vi "Dequeue Cmds From Nodes.vi"(6 "Ready For Output?":bool, 7 "NumNodes":u8=1, 8 "error in":errorcluster, 11 "Communication FIFOs":T2) -> (0 "error out":errorcluster, 1 "Cmd Received Valid":bool, 2 "Cmd Received":T1, 5 "Current Node":u8)   [LabVIEW 2014, in "IO Node Logic Template.lvlib"]
uses:
  IO Node Logic Template.lvlib
  Controls/All Nodes Resources.ctl
  Node/Controls/NodeResources FIFOs.ctl
  Node/Controls/Node_Command_Sent.ctl
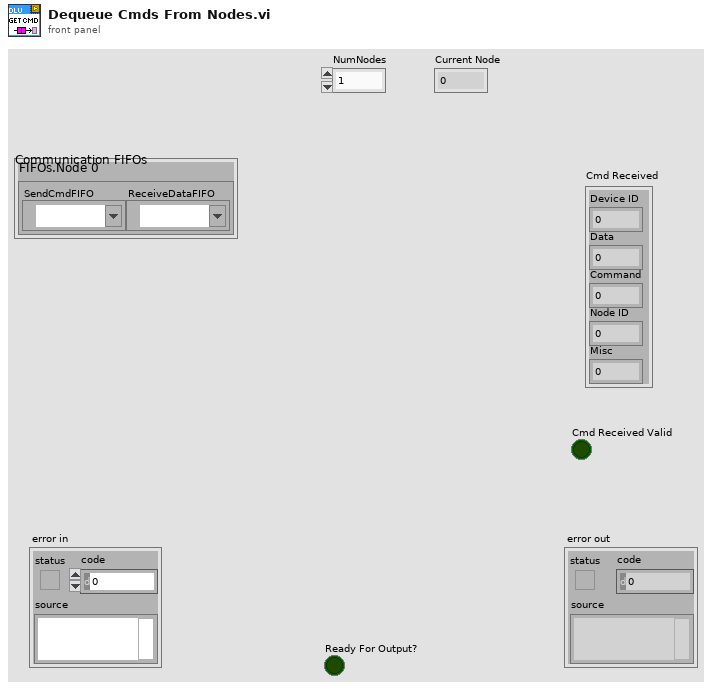
[diagram p1: front panel]
types:
  T1 = typedef "Node_Command_Sent.ctl" = cluster{"Device ID":u8, "Data":u64, "Command":u8, "Node ID":u8, "Misc":u8}
  T2 = typedef "IO Node Logic Template.lvlib/All Nodes Resources.ctl" = cluster{"FIFOs.Node 0":T3}
  T3 = typedef "IO Node Logic Template.lvlib/NodeResources FIFOs.ctl" = cluster{"SendCmdFIFO":refnum<k21>, "ReceiveDataFIFO":refnum<k21>}
  T4 = cluster{"Channel ID":u8, "Data":u64, "Command":u8, "Sender Address":u8, "Misc":u8}
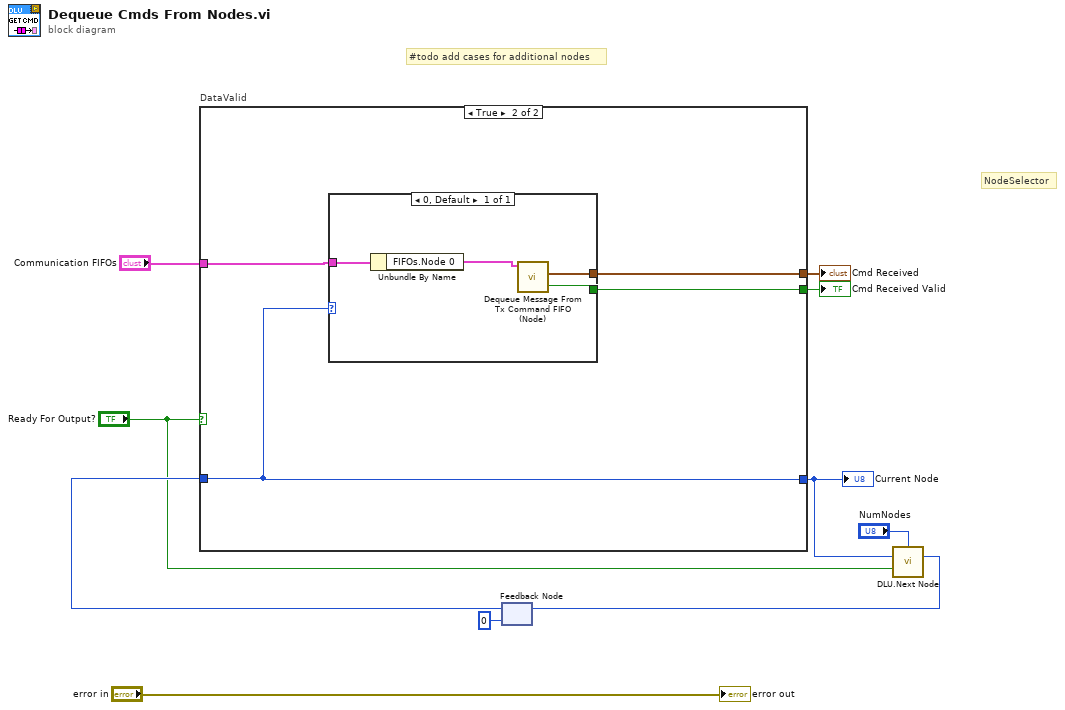
[diagram p0: block diagram]
diagram:
  # "#todo add cases for additional nodes"
  # "NodeSelector"
  n1 = feedback #1(u8 0 ("Next Node")) -> (w7:u8)
  n2 = case "DataValid" shown="True" "Ready For Output?" {
    tunnel: w7 -> [w11 w12]
    tunnel: "Communication FIFOs" -> [_ w15]
    tunnel: [_ w14] -> w3
    tunnel: [_ w13] -> w2
    tunnel: [w11 w12] -> w6
    frame False {
    }
    frame True {
      n3 = case shown="0, Default" w12 {
        tunnel: w15 -> [w19]
        tunnel: [w18] -> w14
        tunnel: [w17] -> w13
        frame 0, Default {
          n4 = Unbundle By Name(w19) -> ("FIFOs.Node 0"=w16:T3)
          n5 = call "Dequeue Message From Tx Command FIFO (Node).vi"("FIFOs: I/O Node"=w16) -> ("Cmd Received Valid"=w17:bool, "Cmd Received"=w18:T4)  [unwired: 7 in, 2 out]
        }
      }
    }
  }
  "Cmd Received" <- w3
  "Cmd Received Valid" <- w2
  "Current Node" <- w6
  n6 = call "DLU.Next Node.vi"("NumNodes"="NumNodes", "Current Node"=w6, "Move to Next Node"="Ready For Output?") -> ("Next Node"=w9:u8)  [unwired: 12 in]
  n7 = feedback-in #1(w9) -> ()
  "error out" <- "error in"
